vi "test-diff-drive-kinematics.vi"() -> (3 "All Passed":bool)   [LabVIEW 2019]
uses:
  <vilib>/Rock Robotics/SystemInterfaces/NetworkCommunication/NetComm_UsageReport_report.vi
  <vilib>/Rock Robotics/WPI/ThirdParty/JAS_Junk/TrajLib/Util_LibraryGlobals.vi
  <vilib>/Rock Robotics/WPI/ThirdParty/JAS_Junk/TrajLib/Trajectory_Library.lvlib
panel:
  out "Passed Test 5":bool
  out "Passed Test 4":bool
  out "Passed Test 3":bool
  out "Passed Test 2":bool
  out "Passed Test 1":bool
  out "Passed Test 0":bool
  # "Diff Drive Kinematic Test"
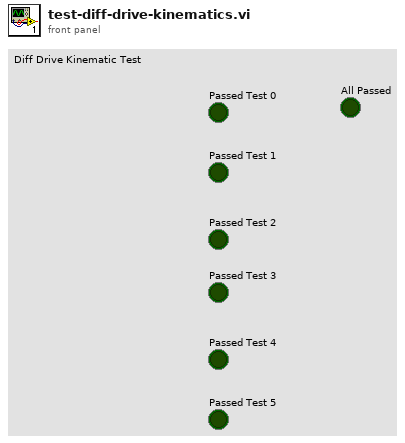
[diagram p1: front panel]
types:
  T1 = typedef "Trajectory_Library.lvlib/CHASSIS_SPEEDS.ctl" = cluster{"vX":dbl, "vY":dbl, "vOmega":dbl}
  T2 = typedef "Trajectory_Library.lvlib/DIFF_DRIVE_KINEMATICS.ctl" = cluster{"TrackWidth_Meters":dbl}
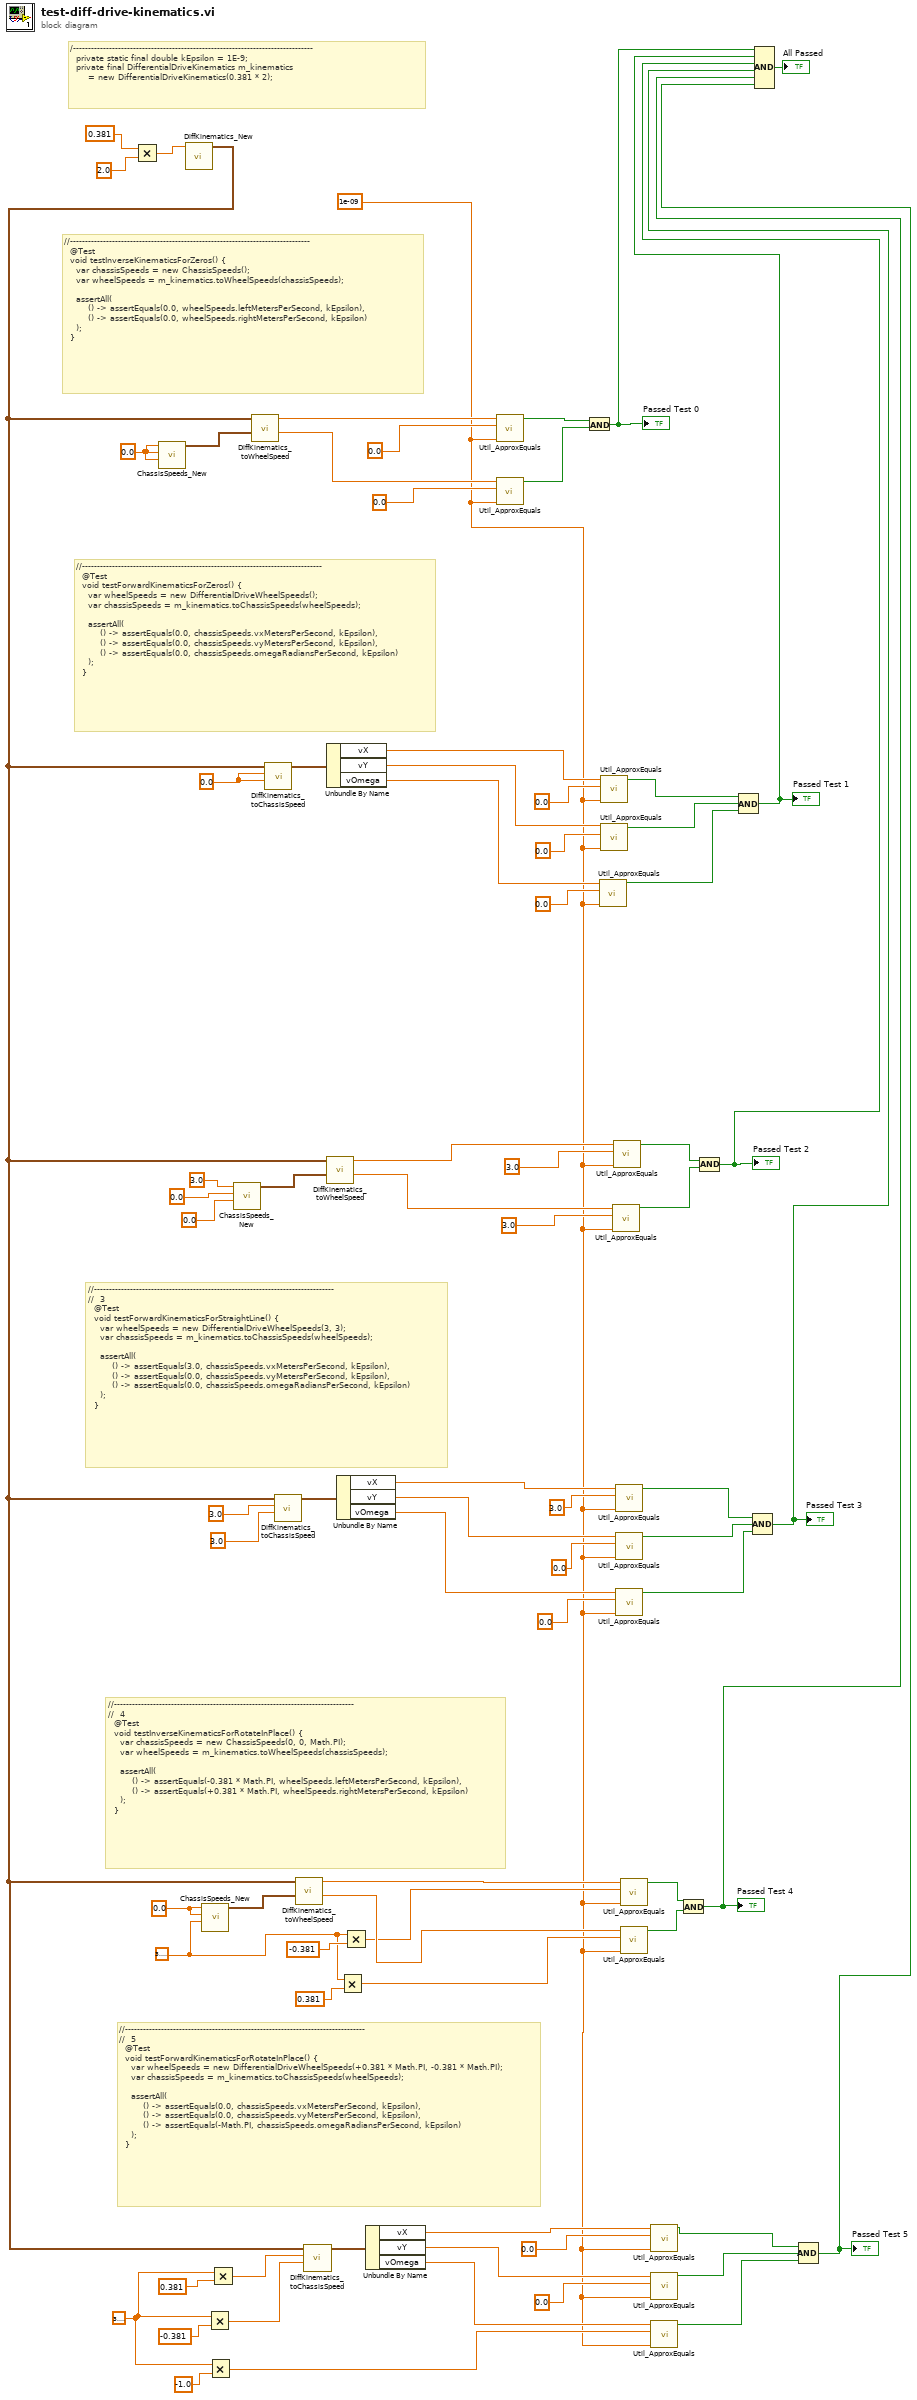
[diagram p0: block diagram]
diagram:
  w1 = 1e-09 ("y")
  w54 = 3.141592653589793
  w62 = 3.141592653589793
  w66 = 0.0 ("vX")
  w75 = 0.0 ("LeftVelocity")
  w77 = 0.0 ("vX")
  # "//--------------------------------------------------------------------------------\n//  5\n  @Test\n  void testForwardKinematicsForRotateInPlace() {\n    var wheelSpeeds = new DifferentialDriveWheelSpeeds(+0.381 * Math.PI, -0.381 * Math.PI);\n    var chassisSpeeds = m_kinematics.toChassisSpeeds(wheelSpeeds);\n\n    assertAll(\n        () -> assertEquals(0.0, chassisSpeeds.vxMetersPerSecond, kEpsilon),\n        () -> assertEquals(0.0, chassisSpeeds.vyMetersPerSecond, kEpsilon),\n        () -> assertEquals(-Math.PI, chassisSpeeds.omegaRadiansPerSecond, kEpsilon)\n    );\n  }"
  # "//--------------------------------------------------------------------------------\n//  4\n  @Test\n  void testInverseKinematicsForRotateInPlace() {\n    var chassisSpeeds = new ChassisSpeeds(0, 0, Math.PI);\n    var wheelSpeeds = m_kinematics.toWheelSpeeds(chassisSpeeds);\n\n    assertAll(\n        () -> assertEquals(-0.381 * Math.PI, wheelSpeeds.leftMetersPerSecond, kEpsilon),\n        () -> assertEquals(+0.381 * Math.PI, wheelSpeeds.rightMetersPerSecond, kEpsilon)\n    );\n  }"
  # "//--------------------------------------------------------------------------------\n//  3\n  @Test\n  void testForwardKinematicsForStraightLine() {\n    var wheelSpeeds = new DifferentialDriveWheelSpeeds(3, 3);\n    var chassisSpeeds = m_kinematics.toChassisSpeeds(wheelSpeeds);\n\n    assertAll(\n        () -> assertEquals(3.0, chassisSpeeds.vxMetersPerSecond, kEpsilon),\n        () -> assertEquals(0.0, chassisSpeeds.vyMetersPerSecond, kEpsilon),\n        () -> assertEquals(0.0, chassisSpeeds.omegaRadiansPerSecond, kEpsilon)\n    );\n  }"
  # "//--------------------------------------------------------------------------------\n  @Test\n  void testForwardKinematicsForZeros() {\n    var wheelSpeeds = new DifferentialDriveWheelSpeeds();\n    var chassisSpeeds = m_kinematics.toChassisSpeeds(wheelSpeeds);\n\n    assertAll(\n        () -> assertEquals(0.0, chassisSpeeds.vxMetersPerSecond, kEpsilon),\n        () -> assertEquals(0.0, chassisSpeeds.vyMetersPerSecond, kEpsilon),\n        () -> assertEquals(0.0, chassisSpeeds.omegaRadiansPerSecond, kEpsilon)\n    );\n  }"
  # "/--------------------------------------------------------------------------------\n  private static final double kEpsilon = 1E-9;\n  private final DifferentialDriveKinematics m_kinematics\n      = new DifferentialDriveKinematics(0.381 * 2);"
  # "//--------------------------------------------------------------------------------\n  @Test\n  void testInverseKinematicsForZeros() {\n    var chassisSpeeds = new ChassisSpeeds();\n    var wheelSpeeds = m_kinematics.toWheelSpeeds(chassisSpeeds);\n\n    assertAll(\n        () -> assertEquals(0.0, wheelSpeeds.leftMetersPerSecond, kEpsilon),\n        () -> assertEquals(0.0, wheelSpeeds.rightMetersPerSecond, kEpsilon)\n    );\n  }"
  n1 = Multiply(x=0.381, y=2.0) -> (x*y=w78:dbl)
  n2 = call <vilib>:"ChassisSpeeds_New.vi"("vAngular"=w77, "vY"=w77, "vX"=w77) -> ("CHASSIS"=w76:T1)  [unwired: 8 in]
  n3 = call <vilib>:"DiffKinematics_New.vi"("TrackWidth_Meters"=w78) -> ("DIFF_DRIVE_KINEMATICS"=w60:T2)  [unwired: 10 in]
  n4 = call <vilib>:"ChassisSpeeds_New.vi"("vAngular"=w62, "vY"=w66, "vX"=w66) -> ("CHASSIS"=w65:T1)  [unwired: 8 in]
  n5 = Multiply(x=w54, y=-0.381) -> (x*y=w56:dbl)
  n6 = Multiply(x=w54, y=-1.0) -> (x*y=w13:dbl)
  n7 = Multiply(x=w54, y=0.381) -> (x*y=w57:dbl)
  n8 = call <vilib>:"ChassisSpeeds_New.vi"("vAngular"=0.0, "vY"=0.0, "vX"=3.0) -> ("CHASSIS"=w73:T1)  [unwired: 8 in]
  n9 = call <vilib>:"DiffKinematics_toWheelSpeed.vi"("CHASSIS Speed"=w76, "DIFF_DRIVE_KINEMATICS"=w60) -> ("RightVelocity"=w45:dbl, "LeftVelocity"=w46:dbl)  [unwired: 8 in]
  n10 = call <vilib>:"DiffKinematics_toChassisSpeed.vi"("RightVelocity"=w75, "LeftVelocity"=w75, "inDIFF_DRIVE_KINEMATICS"=w60) -> ("CHASSIS Speed"=w74:T1)  [unwired: 8 in]
  n11 = call <vilib>:"DiffKinematics_toChassisSpeed.vi"("RightVelocity"=3.0, "LeftVelocity"=3.0, "inDIFF_DRIVE_KINEMATICS"=w60) -> ("CHASSIS Speed"=w68:T1)  [unwired: 8 in]
  n12 = call <vilib>:"DiffKinematics_toWheelSpeed.vi"("CHASSIS Speed"=w65, "DIFF_DRIVE_KINEMATICS"=w60) -> ("RightVelocity"=w5:dbl, "LeftVelocity"=w4:dbl)  [unwired: 8 in]
  n13 = call <vilib>:"DiffKinematics_toChassisSpeed.vi"("RightVelocity"=w56, "LeftVelocity"=w57, "inDIFF_DRIVE_KINEMATICS"=w60) -> ("CHASSIS Speed"=w61:T1)  [unwired: 8 in]
  n14 = Unbundle By Name(w74) -> ("vX"=w40:dbl, "vY"=w39:dbl, "vOmega"=w38:dbl)
  n15 = call <vilib>:"DiffKinematics_toWheelSpeed.vi"("CHASSIS Speed"=w73, "DIFF_DRIVE_KINEMATICS"=w60) -> ("RightVelocity"=w29:dbl, "LeftVelocity"=w31:dbl)  [unwired: 8 in]
  n16 = Unbundle By Name(w68) -> ("vX"=w22:dbl, "vY"=w21:dbl, "vOmega"=w20:dbl)
  n17 = Multiply(x=w62, y=0.381) -> (x*y=w2:dbl)
  n18 = Multiply(x=w62, y=-0.381) -> (x*y=w3:dbl)
  n19 = Unbundle By Name(w61) -> ("vX"=w16:dbl, "vY"=w15:dbl, "vOmega"=w14:dbl)
  n20 = call "Util_ApproxEquals.vi"("Tolerance"=w1, "Value 2"=0.0 ("y"), "Value 1"=w46) -> ("ApproxEquals"=w42:bool)  [unwired: 8 in]
  n21 = call "Util_ApproxEquals.vi"("Tolerance"=w1, "Value 2"=0.0 ("y"), "Value 1"=w45) -> ("ApproxEquals"=w41:bool)  [unwired: 8 in]
  n22 = And(x=w42, y=w41) -> (x .and. y?=w53:bool)
  "Passed Test 0" <- w53
  n23 = call "Util_ApproxEquals.vi"("Tolerance"=w1, "Value 2"=0.0 ("y"), "Value 1"=w38) -> ("ApproxEquals"=w32:bool)  [unwired: 8 in]
  n24 = call "Util_ApproxEquals.vi"("Tolerance"=w1, "Value 2"=0.0 ("y"), "Value 1"=w40) -> ("ApproxEquals"=w34:bool)  [unwired: 8 in]
  n25 = call "Util_ApproxEquals.vi"("Tolerance"=w1, "Value 2"=0.0 ("y"), "Value 1"=w39) -> ("ApproxEquals"=w33:bool)  [unwired: 8 in]
  n26 = call "Util_ApproxEquals.vi"("Tolerance"=w1, "Value 2"=3.0 ("y"), "Value 1"=w29) -> ("ApproxEquals"=w26:bool)  [unwired: 8 in]
  n27 = call "Util_ApproxEquals.vi"("Tolerance"=w1, "Value 2"=3.0 ("y"), "Value 1"=w31) -> ("ApproxEquals"=w27:bool)  [unwired: 8 in]
  n28 = call "Util_ApproxEquals.vi"("Tolerance"=w1, "Value 2"=3.0 ("y"), "Value 1"=w22) -> ("ApproxEquals"=w25:bool)  [unwired: 8 in]
  n29 = call "Util_ApproxEquals.vi"("Tolerance"=w1, "Value 2"=0.0 ("y"), "Value 1"=w21) -> ("ApproxEquals"=w24:bool)  [unwired: 8 in]
  n30 = call "Util_ApproxEquals.vi"("Tolerance"=w1, "Value 2"=0.0 ("y"), "Value 1"=w20) -> ("ApproxEquals"=w23:bool)  [unwired: 8 in]
  n31 = call "Util_ApproxEquals.vi"("Tolerance"=w1, "Value 2"=w3, "Value 1"=w4) -> ("ApproxEquals"=w7:bool)  [unwired: 8 in]
  n32 = call "Util_ApproxEquals.vi"("Tolerance"=w1, "Value 2"=w2, "Value 1"=w5) -> ("ApproxEquals"=w6:bool)  [unwired: 8 in]
  n33 = call "Util_ApproxEquals.vi"("Tolerance"=w1, "Value 2"=0.0 ("y"), "Value 1"=w16) -> ("ApproxEquals"=w10:bool)  [unwired: 8 in]
  n34 = call "Util_ApproxEquals.vi"("Tolerance"=w1, "Value 2"=0.0 ("y"), "Value 1"=w15) -> ("ApproxEquals"=w9:bool)  [unwired: 8 in]
  n35 = call "Util_ApproxEquals.vi"("Tolerance"=w1, "Value 2"=w13, "Value 1"=w14) -> ("ApproxEquals"=w8:bool)  [unwired: 8 in]
  n36 = Compound Arithmetic op=AND(w7, w6) -> (w49:bool)
  "Passed Test 4" <- w49
  n37 = Compound Arithmetic op=AND(w27, w26) -> (w51:bool)
  "Passed Test 2" <- w51
  n38 = Compound Arithmetic op=AND(w34, w33, w32) -> (w52:bool)
  "Passed Test 1" <- w52
  n39 = Compound Arithmetic op=AND(w25, w24, w23) -> (w50:bool)
  "Passed Test 3" <- w50
  n40 = Compound Arithmetic op=AND(w10, w9, w8) -> (w48:bool)
  "Passed Test 5" <- w48
  n41 = Compound Arithmetic op=AND(w53, w52, w51, w50, w49, w48) -> (→"All Passed":bool)
